vi "Done--Const.vi"() -> (3 "Done Message":string)   [LabVIEW 2017, in "Communications Library.lvlib"]
uses:
  Communications Library.lvlib
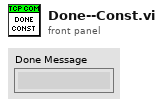
[diagram p1: front panel]
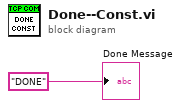
[diagram p0: block diagram]
diagram:
  "Done Message" <- "DONE" ("data in")
